vi "Array Deduplication.vi"   [LabVIEW 2020]
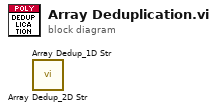
[diagram p0: block diagram]
diagram:
  n1 = call "Array Dedup_2D Str.vi"() -> ()  [unwired: 10 in, 2 out]
  n2 = call "Array Dedup_1D Str.vi"() -> ()  [unwired: 10 in, 2 out]
